vi "SUMM.vi"(9 "Y":i32, 10 "X":i32) -> (0 "Y":i32, 1 "Y+1":i32, 2 "X+1":i32, 3 "X":i32, 4 "Y-1":i32, 5 "X-1":i32)   [LabVIEW 2016]
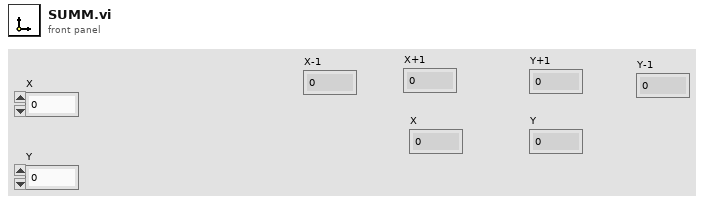
[diagram p1: front panel]
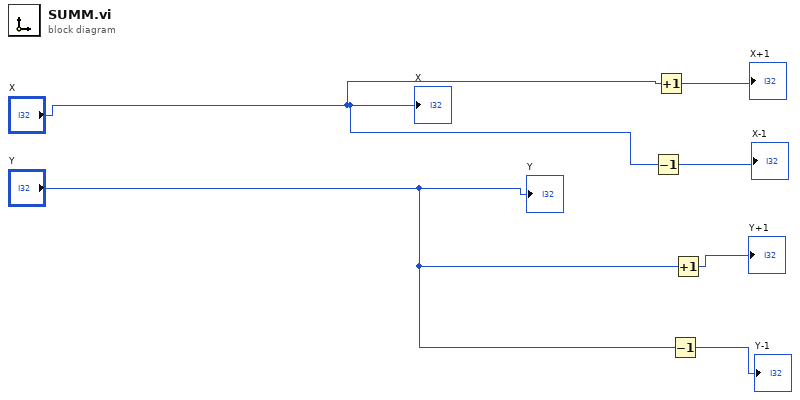
[diagram p0: block diagram]
diagram:
  n1 = Decrement(x="X") -> (x-1=→"X-1":i32)
  n2 = Increment(x="X") -> (x+1=→"X+1":i32)
  n3 = Decrement(x="Y") -> (x-1=→"Y-1":i32)
  n4 = Increment(x="Y") -> (x+1=→"Y+1":i32)
  "X" <- "X"
  "Y" <- "Y"
